vi "Enqueue_Queue_Array.vi"(6 "Prioty":bool, 8 "error in (no error)":errorcluster, 9 "Data":variant[](array[variant]), 10 "Command":string[](array[string]), 11 "queue In":refnum<queue>) -> (0 "error out":errorcluster, 3 "queue Out":refnum<queue>)   [LabVIEW 2014, in "Queue_Library.lvlib"]
uses:
  Queue_Library.lvlib
  TypeDef.ctl
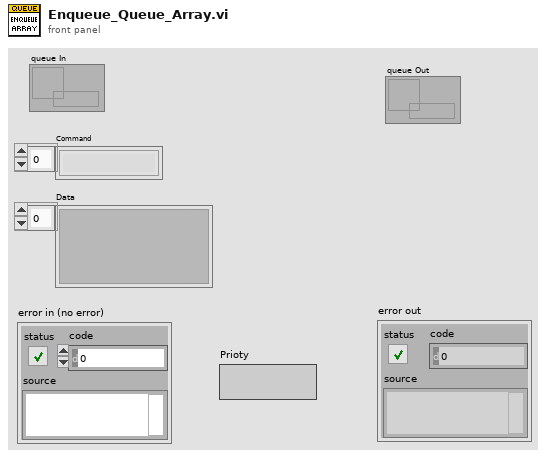
[diagram p1: front panel]
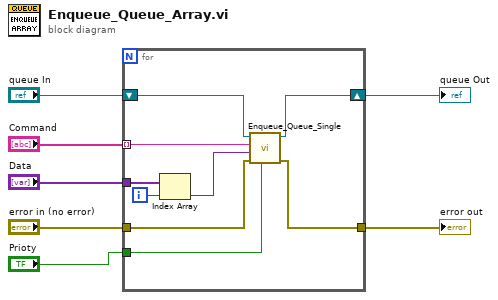
[diagram p0: block diagram]
diagram:
  n1 = for {
    shift-right: [w15] -> w6
    shift-left: "queue In" -> [w16]
    tunnel: [w14] -> w5
    tunnel: "error in (no error)" -> [w13]
    tunnel: "Prioty" -> [w12]
    tunnel: "Command" -> [w11] mode=indexing
    tunnel: "Data" -> [w10]
    i -> [w9]
    n2 = Index Array(array=w10, index=w9) -> (element=w8:variant)
    n3 = call "Enqueue_Queue_Single.vi"("Prioty"=w12, "error in (no error)"=w13, "Data"=w8, "Command"=w11, "queue In"=w16) -> ("error out"=w14:errorcluster, "queue Out"=w15:refnum<queue>)  [unwired: 5 in]
  }
  "error out" <- w5
  "queue Out" <- w6
